vi "Test.vi"(8 "error in (no error)":errorcluster, 11 "LogDB in":refnum<class "LogDB.lvclass">) -> (0 "error out":errorcluster, 2 "Pass?":bool, 3 "LogDB out":refnum<class "LogDB.lvclass">)   [LabVIEW 2020, in "LogDB.lvclass"]
uses:
  LogDB.lvclass
  Base Decorator/Base Decorator.lvclass
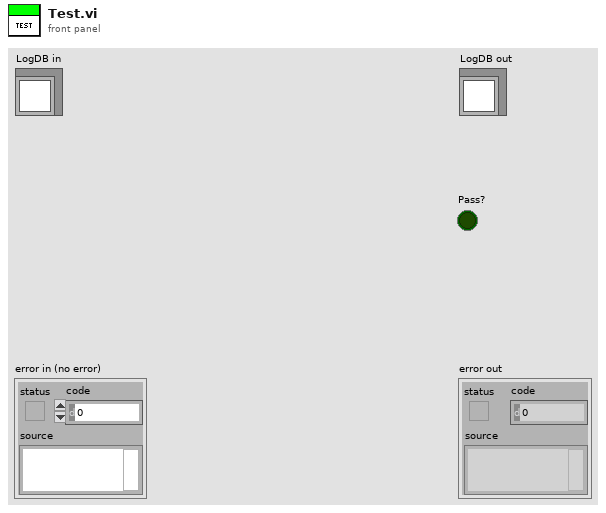
[diagram p1: front panel]
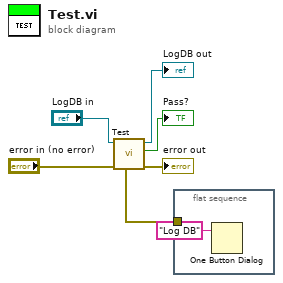
[diagram p0: block diagram]
diagram:
  n1 = call-parent "Test.vi"("error in (no error)"="error in (no error)", "Base Decorator in"="LogDB in") -> ("error out"=w1:errorcluster, "Pass?"=→"Pass?":bool, "Base Decorator out"=→"LogDB out":refnum<class "LogDB.lvclass">)  [unwired: 7 in]
  "error out" <- w1
  n2 = flat-sequence {
    tunnel: w1 -> [_]
    frame #0 {
      n3 = One Button Dialog(message="Log DB") -> ()  [unwired: 1 in, 1 out]
    }
  }
